vi "Send move to stages.vi"(8 "error in (no error)":errorcluster, 11 "ImageStack in":refnum<class "ImageStack.lvclass">) -> (0 "error out":errorcluster, 3 "ImageStack out":refnum<class "ImageStack.lvclass">)   [LabVIEW 2012, in "ImageStack.lvclass"]
uses:
  ImageStack.lvclass
  <vilib>/Distrio/Murmex/GenericMessage/GenericMessage.lvclass
  ImageStack.lvclass/ImageStack.ctl
  <vilib>/Distrio/Murmex/Message/Message.lvclass
  <vilib>/Distrio/Murmex/Murmex/Murmex.lvclass
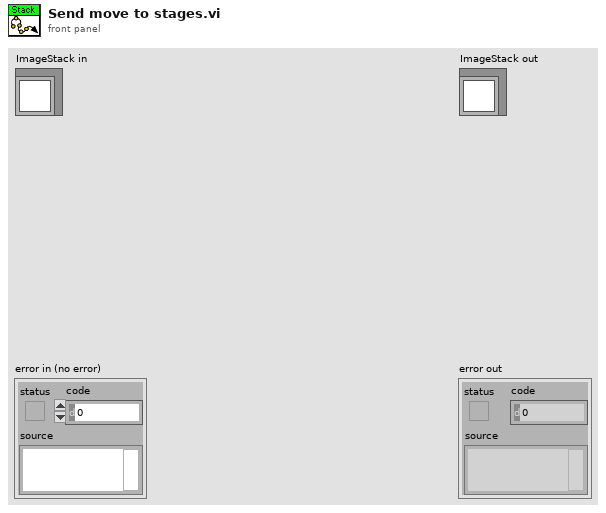
[diagram p1: front panel]
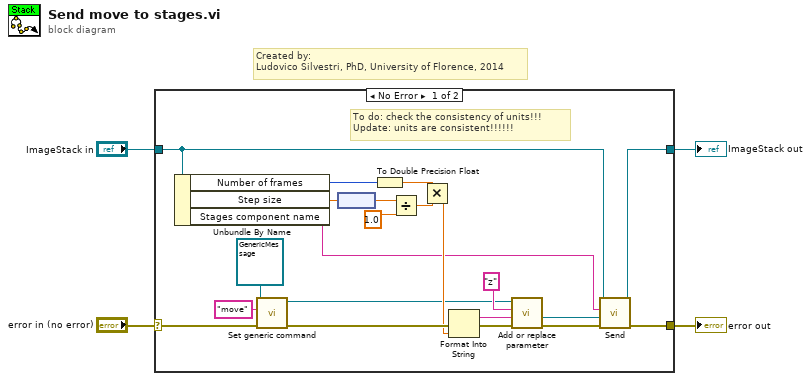
[diagram p0: block diagram]
diagram:
  # "Created by:\nLudovico Silvestri, PhD, University of Florence, 2014"
  n1 = case shown="No Error" "error in (no error)" {
    selector: "error in (no error)" -> [w23 w27]
    tunnel: [w9 w27] -> w3
    tunnel: [w7 w26] -> w1
    tunnel: "ImageStack in" -> [w8 w26]
    frame No Error {
      # "To do: check the consistency of units!!!\nUpdate: units are consistent!!!!!!"
      n2 = Unbundle By Name(w8) -> ("Number of frames"=w18:u16, "Step size"=w22:dbl[unit], "Stages component name"=w5:string)
      n3 = call <vilib>:"Set generic command.vi"("error in (no error)"=w23, "generic command"="move" ("command string"), "GenericMessage in"=refnum<class "GenericMessage.lvclass"> refnum ("Murmex.lvlib:GenericMessage")) -> ("error out"=w16:errorcluster, "GenericMessage out"=w11:refnum<class "GenericMessage.lvclass">)  [unwired: 7 in]
      n4 = node(w22) -> (w21:dbl)
      n5 = To Double Precision Float(number=w18) -> (double precision float=w17:dbl)
      n6 = Divide(x=w21, y=1.0) -> (x/y=w19:dbl)
      n7 = Multiply(x=w17, y=w19) -> (x*y=w15:dbl)
      n8 = Format Into String(error in=w16, w15) -> (resulting string=w13:string, error out=w14:errorcluster)  [unwired: 2 in]
      n9 = call <vilib>:"Add or replace parameter.vi"("error in (no error)"=w14, "value"=w13, "name"="z", "Message in"=w11) -> ("error out"=w10:errorcluster, "Message out"=w6:refnum<class "GenericMessage.lvclass">)  [unwired: 6 in]
      n10 = call <vilib>:"Send.vi"("error in (no error)"=w10, "Message"=w6, "recipient"=w5, "Murmex in"=w8) -> ("error out"=w9:errorcluster, "Murmex out"=w7:refnum<class "ImageStack.lvclass">)  [unwired: 6 in]
    }
    frame Error {
    }
  }
  "error out" <- w3
  "ImageStack out" <- w1
